vi "FlatToRichnixnet_grpc_ConvertFramesToByteArraySinglePointResponse.vi"(5 "OutputClusterType":T1, 11 "InputCluster":T2) -> (3 "OutputCluster":T1)   [LabVIEW 2025, in "grpc-xnet_client.lvlib"]
uses:
  grpc-xnet_client.lvlib
  nixnet_grpc_ConvertFramesToByteArraySinglePointResponse_Flat.ctl
  nixnet_grpc_ConvertFramesToByteArraySinglePointResponse.ctl
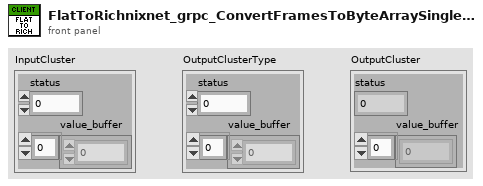
[diagram p1: front panel]
types:
  T1 = typedef "grpc-xnet_client.lvlib/nixnet_grpc_ConvertFramesToByteArraySinglePointResponse.ctl" = cluster{"status":i32, "value_buffer":u8[]}
  T2 = typedef "grpc-xnet_client.lvlib/nixnet_grpc_ConvertFramesToByteArraySinglePointResponse_Flat.ctl" = cluster{"status":i32, "value_buffer":u8[]}
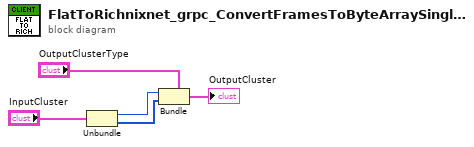
[diagram p0: block diagram]
diagram:
  n1 = Unbundle "Unbundle"("InputCluster") -> ("status"=w2:i32, "value_buffer"=w1:u8[])
  n2 = Bundle "Bundle"(cluster="OutputClusterType", "status"=w2, "value_buffer"=w1) -> (→"OutputCluster":T1)
